vi "HandleDoubleSolenoid.vi"(7 "InitState":T1=enum."Middle", 11 "Toggle?":bool) -> ()   [LabVIEW 2013]
uses:
  DoubleSolenoidAction.ctl
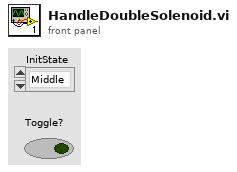
[diagram p1: front panel]
types:
  T1 = typedef "DoubleSolenoidAction.ctl" = enum16{"Init", "Middle", "In", "Out"}
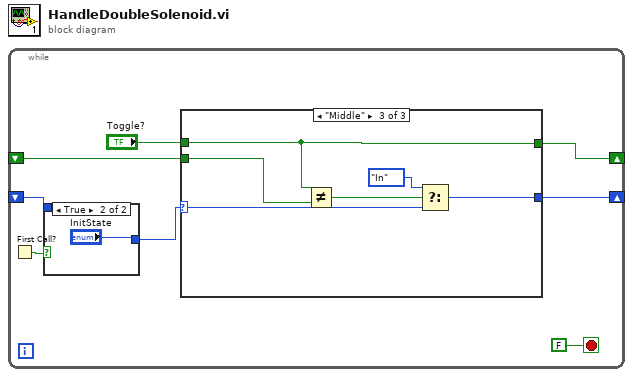
[diagram p0: block diagram]
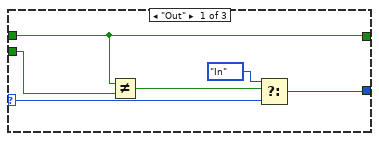
[diagram p3: hidden frame]
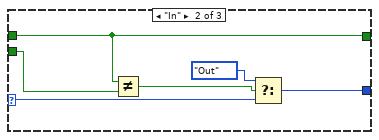
[diagram p4: hidden frame]
diagram:
  n1 = while {
    shift-right: [w7] -> _
    shift-left: _ -> [w4]
    shift-right: [w2] -> _
    shift-left: _ -> [w1]
    stop <- FALSE stop-if-true
    n2 = First Call?() -> (First Call?: T/F=w6:bool)
    n3 = case shown="True" w6 {
      tunnel: [w9 "InitState"] -> w5
      tunnel: w4 -> [w9 _]
      frame False {
      }
      frame True {
      }
    }
    n4 = case shown="\"Middle\"" w5 {
      selector: w5 -> [w14 w20 w28]
      tunnel: [w15 w21 w27] -> w7
      tunnel: [w11 w18 w25] -> w2
      tunnel: "Toggle?" -> [w11 w18 w25]
      tunnel: w1 -> [w12 w17 w24]
      frame "Out" {
        n5 = Not Equal?(x=w11, y=w12) -> (x != y?=w13:bool)
        n6 = Select(t=DoubleSolenoidAction."In", s=w13, f=w14) -> (s? t:f=w15:T1)
      }
      frame "In" {
        n7 = Not Equal?(x=w18, y=w17) -> (x != y?=w19:bool)
        n8 = Select(t=DoubleSolenoidAction."Out", s=w19, f=w20) -> (s? t:f=w21:T1)
      }
      frame "Middle" {
        n9 = Not Equal?(x=w25, y=w24) -> (x != y?=w23:bool)
        n10 = Select(t=DoubleSolenoidAction."In", s=w23, f=w28) -> (s? t:f=w27:T1)
      }
    }
  }
